vi "Write Control Tags.vi"(7 "Sequence Control":T1, 10 "Prameter allocation in":T2, 11 "Sequencer Module runtime in":refnum<class "Sequencer Module runtime.lvclass">) -> (2 "Parameter allocation out":T2, 3 "Sequencer Module runtime out":refnum<class "Sequencer Module runtime.lvclass">)   [LabVIEW 2015, in "Sequencer Module runtime.lvclass"]
uses:
  Sequencer Module runtime.lvclass
  <vilib>/NI/Tag Bus/table/data table.ctl
  Sequencer Control.ctl
  Sequencer Module runtime.lvclass/Sequencer Module runtime.ctl
  <vilib>/NI/Tag Bus/table/data polymorphs/write one/write Boolean.vi
  <vilib>/NI/Tag Bus/table/data polymorphs/write one/write I32.vi
  <vilib>/NI/Tag Bus/table/data table.lvlib
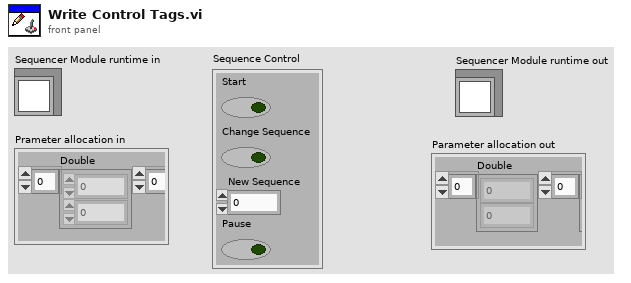
[diagram p1: front panel]
types:
  T1 = typedef "Sequencer Module runtime.lvclass/Sequencer Control.ctl" = cluster{"Start":bool, "Change Sequence":bool, "New Sequence":i32, "Pause":bool}
  T2 = typedef "tag bus.lvlib/data table.lvlib/data table.ctl" = cluster{"Double":dbl[], "Single":sgl[], "I64":i64[], "I32":i32[], "I16":i16[], "I8":i8[], "U64":u64[], "U32":u32[], "U16":u16[], "U8":u8[], "Boolean":bool[], "String":string[], "Array of Double":cluster{"DBL Array":dbl[]}[], "Array of Single":cluster{"SGL Array":sgl[]}[], "Array of I64":cluster{"I64 Array":i64[]}[], "Array of I32":cluster{"I32 Array":i32[]}[], "Array of I16":cluster{"I16 Array":i16[]}[], "Array of I8":cluster{"I8 Array":i8[]}[], "Array of U64":cluster{"U64 Array":u64[]}[], "Array of U32":cluster{"U32 Array":u32[]}[], "Array of U16":cluster{"U16 Array":u16[]}[], "Array of U8":cluster{"U8 Array":u8[]}[], "Array of Boolean":cluster{"Boolean Array":bool[]}[], "Array of String":cluster{"String Array":string[]}[]}
  T3 = typedef "Sequencer Module runtime.lvclass/Sequencer Control Index.ctl" = cluster{"Start":i32, "Change Sequence":i32, "New Sequence":i32, "Pause":i32}
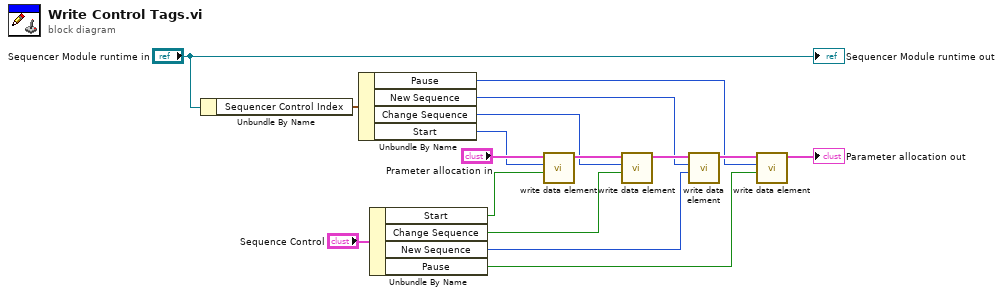
[diagram p0: block diagram]
diagram:
  n1 = Unbundle By Name("Sequencer Module runtime in") -> ("Sequencer Control Index"=w15:T3)
  n2 = Unbundle By Name(w15) -> ("Pause"=w10:i32, "New Sequence"=w1:i32, "Change Sequence"=w2:i32, "Start"=w3:i32)
  n3 = Unbundle By Name("Sequence Control") -> ("Start"=w9:bool, "Change Sequence"=w8:bool, "New Sequence"=w7:i32, "Pause"=w5:bool)
  n4 = call-poly <vilib>:"write data element.vi"("value"=w9, "index"=w3, "data table in"="Prameter allocation in") -> ("data table out"=w13:T2)  [unwired: 8 in]
  n5 = call-poly <vilib>:"write data element.vi"("value"=w8, "index"=w2, "data table in"=w13) -> ("data table out"=w12:T2)  [unwired: 8 in]
  n6 = call-poly <vilib>:"write data element.vi"("value"=w7, "index"=w1, "data table in"=w12) -> ("data table out"=w11:T2)  [unwired: 8 in]
  n7 = call-poly <vilib>:"write data element.vi"("value"=w5, "index"=w10, "data table in"=w11) -> ("data table out"=→"Parameter allocation out":T2)  [unwired: 8 in]
  "Sequencer Module runtime out" <- "Sequencer Module runtime in"
